vi "ClassImplementsMethod.vi"(8 "error in (no error)":errorcluster, 10 "Method Name":string, 11 "Class Refnum":refnum<vi>) -> (0 "error out":errorcluster, 1 "Path":path, 2 "Implements method?":bool, 3 "Class Refnum out":refnum<vi>)   [LabVIEW 2017, in "DynamicDispatchImplementationWalker.lvlib"]
uses:
  DynamicDispatchImplementationWalker.lvlib
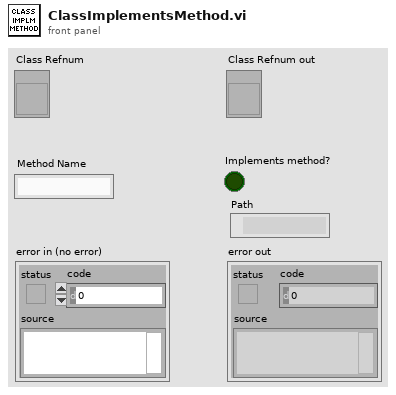
[diagram p1: front panel]
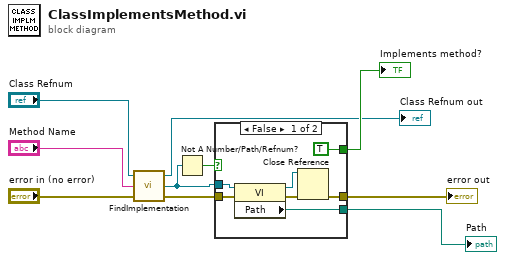
[diagram p0: block diagram]
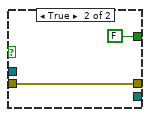
[diagram p2: hidden frame]
diagram:
  n1 = call "FindImplementation.vi"("error in (no error)"="error in (no error)", "Method Name"="Method Name", "Class Refnum"="Class Refnum") -> ("error out"=w5:errorcluster, "VI Reference"=w6:refnum<vi>, "Class out"=→"Class Refnum out":refnum<vi>)
  n2 = Not A Number/Path/Refnum?(number/path/refnum=w6) -> (NaN/Path/Refnum?=w9:bool)
  n3 = case shown="False" w9 {
    tunnel: [w17 w19] -> w10
    tunnel: w5 -> [w12 w19]
    tunnel: w6 -> [w15 _]
    tunnel: [TRUE FALSE] -> w8
    tunnel: [w11 _] -> w1
    frame False {
      n4 = property class="VI"(reference=w15, error in=w12) -> (reference out=w14:refnum<vi>, error out=w13:errorcluster, "Path"=w11:path)
      n5 = Close Reference(reference=w14, error in (no error)=w13) -> (error out=w17:errorcluster)
    }
    frame True {
    }
  }
  "error out" <- w10
  "Implements method?" <- w8
  "Path" <- w1
